vi "destroyEvent.vi"(8 "error in (no error)":errorcluster, 11 "Handler.UserEvent in":refnum<class "Handler.UserEvent.lvclass">) -> (0 "error out":errorcluster, 3 "Handler.UserEvent out":refnum<class "Handler.UserEvent.lvclass">)   [LabVIEW 2017, in "Error Log.lvlib" / "Handler.UserEvent.lvclass"]
uses:
  Handler.UserEvent.lvclass
  Handler.UserEvent.lvclass/Handler.UserEvent.ctl
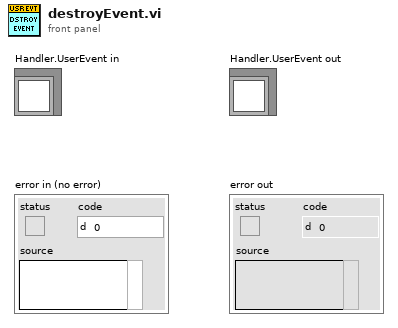
[diagram p1: front panel]
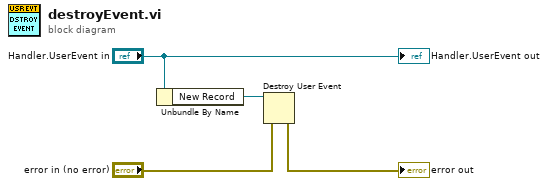
[diagram p0: block diagram]
diagram:
  n1 = Unbundle By Name("Handler.UserEvent in") -> ("New Record"=w1:refnum<user-event>)
  n2 = Destroy User Event(user event=w1, error in="error in (no error)") -> (error out=→"error out":errorcluster)
  "Handler.UserEvent out" <- "Handler.UserEvent in"
